vi "write_wavenumbers_waveforms_2_CSV.vi"(7 "format (%.3f)":string="%.3f", 8 "error in (no error)":errorcluster, 9 "Wavenumber Array":dbl[](array[numeric])=[0.0, 1.0, 2.0, 3.0, 4.0, 5.0, 6.0, 7.0, 8.0, 9.0, 10.0], 10 "Waveform Array":waveform(dbl)[](array[waveform]), 11 "file path (dialog if empty)":path) -> (0 "error out":errorcluster)   [LabVIEW 2020]
uses:
  <vilib>/Waveform/WDTOps.llb/WDT Get Waveform Time Array DBL.vi
  <vilib>/Utility/file.llb/Write Delimited Spreadsheet (DBL).vi
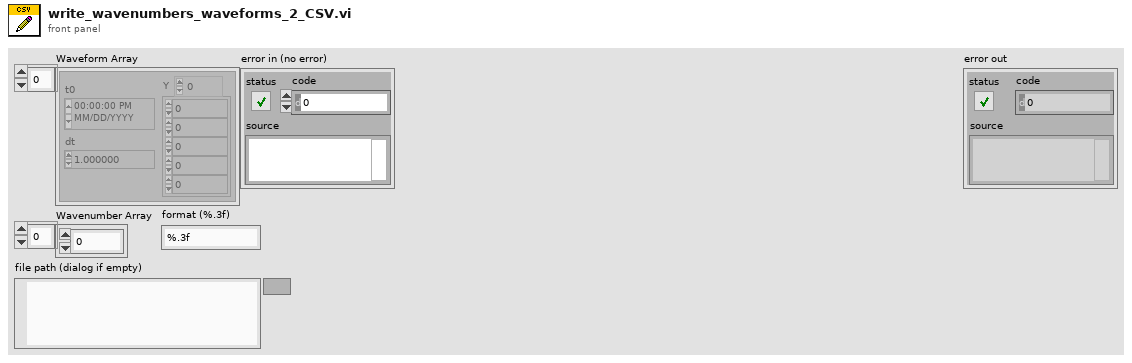
[diagram p1: front panel]
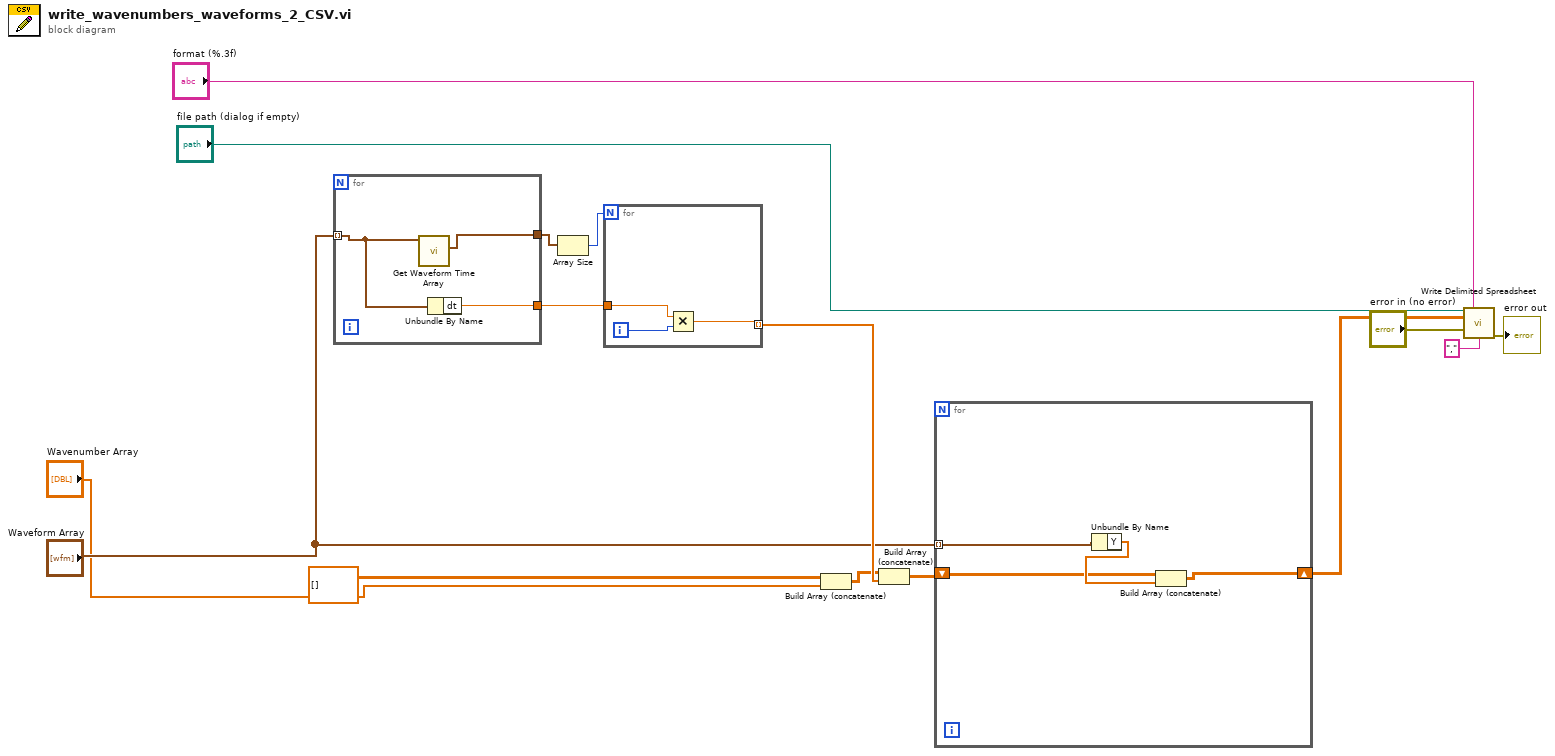
[diagram p0: block diagram]
diagram:
  n1 = for {
    tunnel: "Waveform Array" -> [w17] mode=indexing
    tunnel: [w18] -> w10
    tunnel: [w16] -> w15
    n2 = call-poly <vilib>:"Get Waveform Time Array.vi"("waveform in"=w17) -> ("X array"=w18:timestamp[])  [unwired: 9 in, 1 out]
    n3 = Unbundle By Name(w17) -> ("dt"=w16:dbl)
  }
  n4 = Array Size(array=w10) -> (size(s)=w9:i32)
  n5 = for {
    N: w9 -> [_]
    tunnel: w15 -> [w20]
    tunnel: [w19] -> w13 mode=indexing
    i -> [w21]
    n6 = Multiply(x=w20, y=w21) -> (x*y=w19:dbl)
  }
  n7 = Build Array (concatenate)(dbl[][] [], "Wavenumber Array") -> (w7:dbl[][])
  n8 = Build Array (concatenate)(w7, w13) -> (w14:dbl[][])
  n9 = for {
    tunnel: "Waveform Array" -> [w24] mode=indexing
    shift-right: [w22] -> w11
    shift-left: w14 -> [w23]
    n10 = Unbundle By Name(w24) -> ("Y"=w25:dbl[])
    n11 = Build Array (concatenate)(w23, w25) -> (w22:dbl[][])
  }
  n12 = call-poly <vilib>:"Write Delimited Spreadsheet.vi"("file path (dialog if empty)"="file path (dialog if empty)", "format (%.3f)"="format (%.3f)", "2D data"=w11, "error in (no error)"="error in (no error)", "delimiter (\\t)"="," ("delimiter (\\t)")) -> ("error out"=→"error out":errorcluster)  [unwired: 9 in, 1 out]
